vi "crane_pressure_view.vi"() -> ()   [LabVIEW 2024]
panel:
  out "l5_ground_pressure":dbl(slide)
  out "l4_ground_pressure":dbl(slide)
  out "l3_ground_pressure":dbl(slide)
  out "l2_ground_pressure":dbl(slide)
  out "l1_ground_pressure":dbl(slide)
  out "error out":errorcluster
  in  "stop":bool
  out "period(Hz)":dbl(knob) scale=0.0..20.0
  out "l5_gp_max":bool
  out "l4_gp_max":bool
  out "l3_gp_max":bool
  out "l2_gp_max":bool
  out "l1_gp_max":bool
  out "r5_gp_max":bool
  out "r4_gp_max":bool
  out "r3_gp_max":bool
  out "r2_gp_max":bool
  out "r1_gp_max":bool
  out "MaxGroundPressure":dbl(graph)
  out "Load_state":cluster{"Load(kg)":dbl, "Load_Height(m)":dbl}(graph)
  out "Angle":T1(graph)
  in  "Load_Height(m)":dbl(slide) scale=0.0..10.0
  in  "Load(ton)":dbl(slide) scale=1.0..2.0
  in  "boom_angle(degree)":dbl(knob) scale=30.0..50.0
  in  "swing_angle(degree)":dbl(knob) scale=0.0..90.0
  out "r5_ground_pressure":dbl(slide) scale=0.0..10.0
  out "r4_ground_pressure":dbl(slide) scale=0.0..10.0
  out "r3_ground_pressure":dbl(slide) scale=0.0..10.0
  out "r2_ground_pressure":dbl(slide) scale=0.0..10.0
  out "r1_ground_pressure":dbl(slide) scale=0.0..10.0
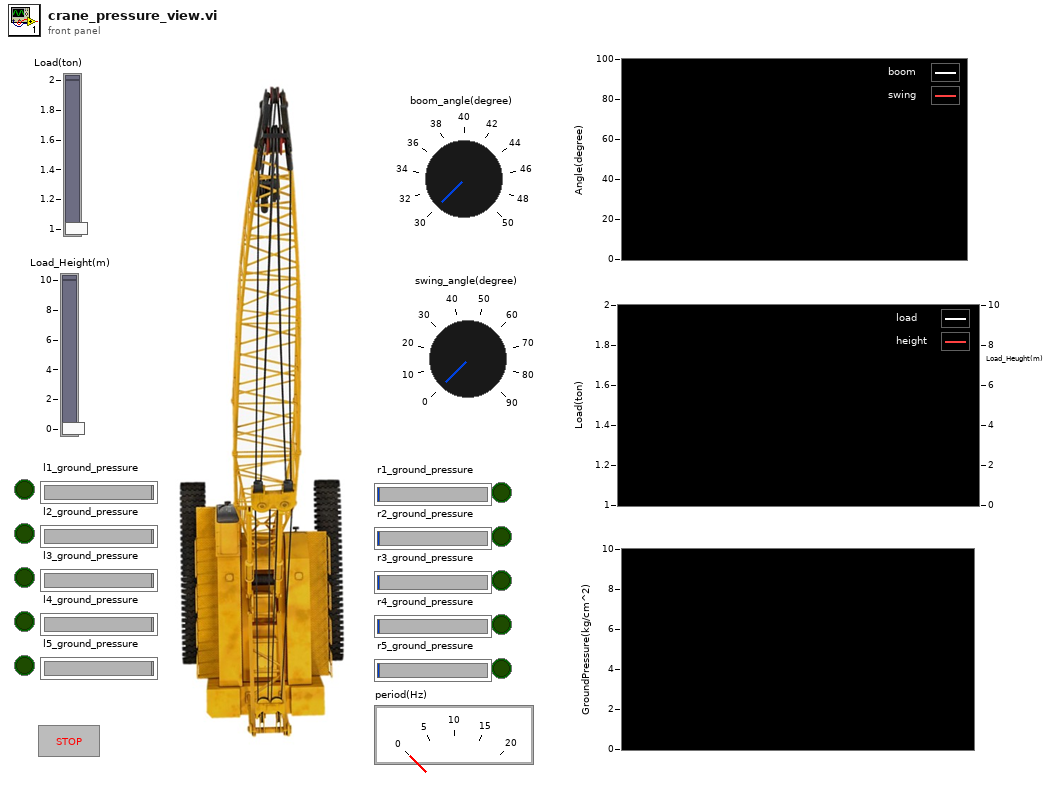
[diagram p1: front panel]
types:
  T1 = cluster{"boom_angle(degree)":dbl, "swing_angle(degree)":dbl}
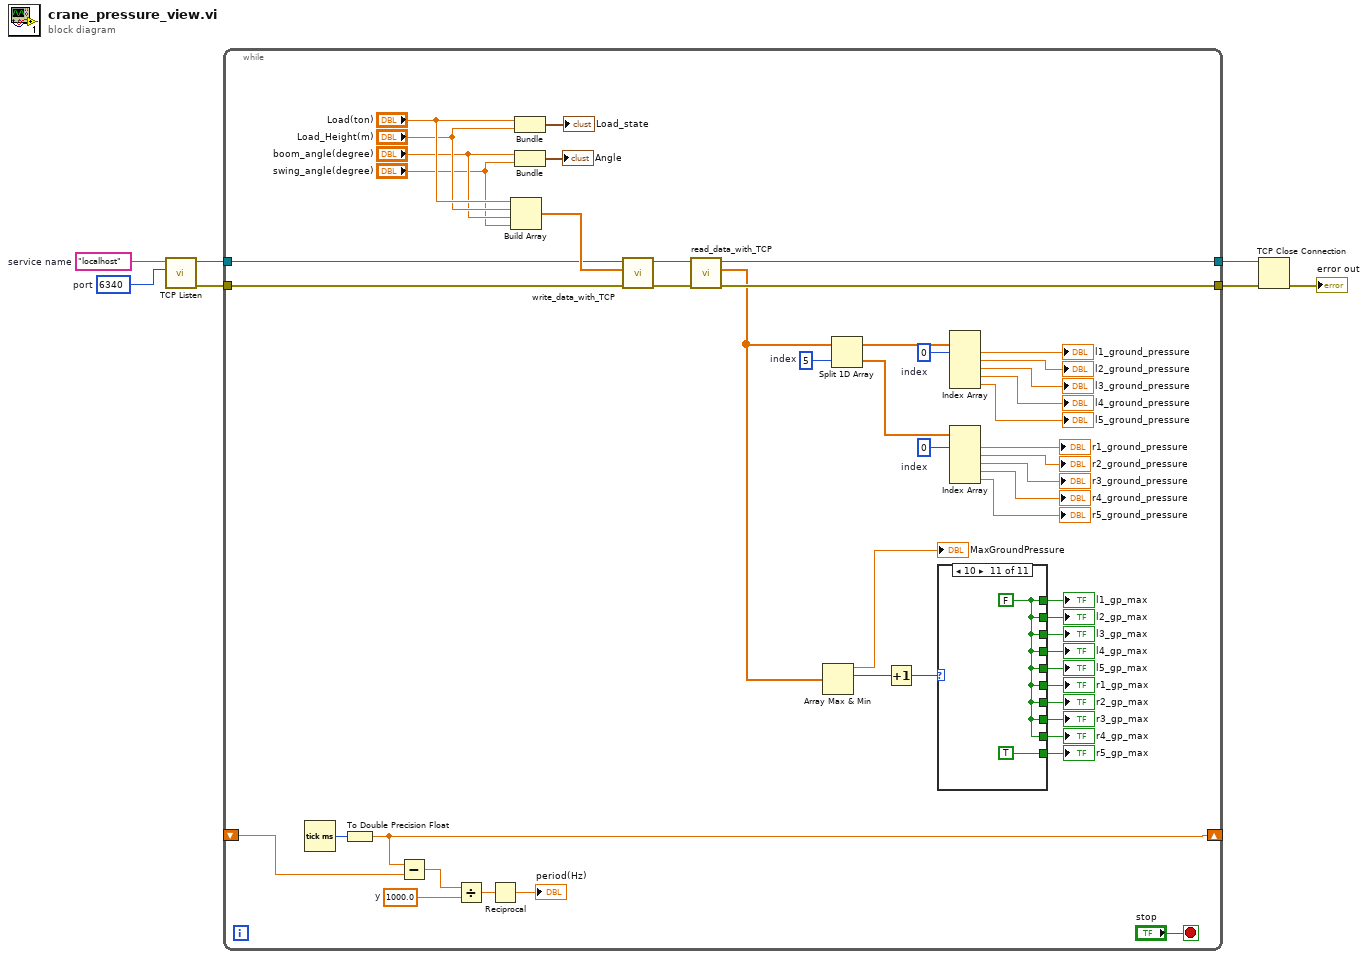
[diagram p0: block diagram]
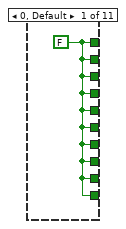
[diagram p2: hidden frame]
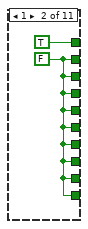
[diagram p3: hidden frame]
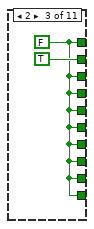
[diagram p4: hidden frame]
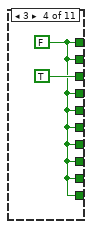
[diagram p5: hidden frame]
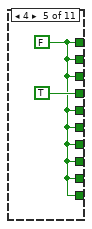
[diagram p6: hidden frame]
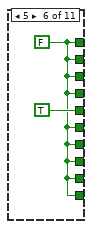
[diagram p7: hidden frame]
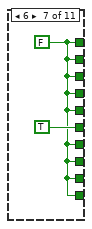
[diagram p8: hidden frame]
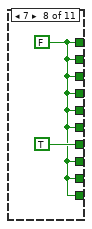
[diagram p9: hidden frame]
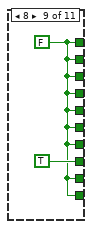
[diagram p10: hidden frame]
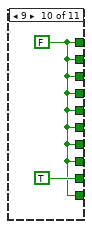
[diagram p11: hidden frame]
diagram:
  w6 = u16 6340  # port
  w7 = "localhost"  # service name
  n1 = call <vilib>:"TCP Listen.vi"("port"=w6, "service name"=w7) -> ("error out"=w4:errorcluster, "connection ID"=w5:refnum<k5>)  [unwired: 5 in, 3 out]
  n2 = while {
    tunnel: w5 -> [w38]
    tunnel: w4 -> [w37]
    tunnel: [w36] -> w3
    tunnel: [w35] -> w2
    shift-right: [w30] -> _
    shift-left: _ -> [w29]
    stop <- "stop" stop-if-true
    w19 = 0  # index
    w21 = 5  # index
    w33 = 1000.0  # y
    w39 = 0  # index
    n3 = Tick Count (ms)() -> (millisecond timer value=w31:u32)
    n4 = To Double Precision Float(number=w31) -> (double precision float=w30:dbl)
    n5 = Subtract(x=w30, y=w29) -> (x-y=w34:dbl)
    n6 = Divide(x=w34, y=w33) -> (x/y=w32:dbl)
    n7 = Reciprocal(x=w32) -> (1/x=→"period(Hz)":dbl)
    n8 = Build Array("Load(ton)", "Load_Height(m)", "boom_angle(degree)", "swing_angle(degree)") -> (w44:dbl[])
    n9 = Bundle("Load(ton)"="Load(ton)", "Load_Height(m)"="Load_Height(m)") -> (→"Load_state":cluster{"Load(ton)":dbl, "Load_Height(m)":dbl})  [unwired: 1 in]
    n10 = Bundle("boom_angle(degree)"="boom_angle(degree)", "swing_angle(degree)"="swing_angle(degree)") -> (→"Angle":T1)  [unwired: 1 in]
    n11 = call "write_data_with_TCP.vi"("error_in"=w37, "data_in"=w44, "TCP_ref_in"=w38) -> ("error_out"=w40:errorcluster, "TCP_ref_out"=w41:refnum<k5>)  [unwired: 7 in]
    n12 = call "read_data_with_TCP.vi"("error_in"=w40, "TCP_ref_in"=w41) -> ("error_out"=w35:errorcluster, "data_out"=w22:dbl[], "TCP_ref_out"=w36:refnum<k5>)  [unwired: 7 in]
    n13 = Array Max & Min(array=w22) -> (max value=→"MaxGroundPressure":dbl, max index (indices)=w47:i32)  [unwired: 2 out]
    n14 = Split 1D Array(array=w22, index=w21) -> (first subarray=w13:dbl[], second subarray=w20:dbl[])
    n15 = Increment(x=w47) -> (x+1=w46:i32)
    n16 = case shown="10" w46 {
      tunnel: [w58 TRUE w61 w63 w65 w67 w69 w71 w73 w75 w77] -> w57
      tunnel: [w58 w59 TRUE w63 w65 w67 w69 w71 w73 w75 w77] -> w56
      tunnel: [w58 w59 w61 TRUE w65 w67 w69 w71 w73 w75 w77] -> w55
      tunnel: [w58 w59 w61 w63 TRUE w67 w69 w71 w73 w75 w77] -> w54
      tunnel: [w58 w59 w61 w63 w65 TRUE w69 w71 w73 w75 w77] -> w53
      tunnel: [w58 w59 w61 w63 w65 w67 TRUE w71 w73 w75 w77] -> w52
      tunnel: [w58 w59 w61 w63 w65 w67 w69 TRUE w73 w75 w77] -> w51
      tunnel: [w58 w59 w61 w63 w65 w67 w69 w71 TRUE w75 w77] -> w50
      tunnel: [w58 w59 w61 w63 w65 w67 w69 w71 w73 TRUE w77] -> w49
      tunnel: [w58 w59 w61 w63 w65 w67 w69 w71 w73 w75 TRUE] -> w48
      frame 0, Default {
        w58 = FALSE
      }
      frame 1 {
        w59 = FALSE
      }
      frame 2 {
        w61 = FALSE
      }
      frame 3 {
        w63 = FALSE
      }
      frame 4 {
        w65 = FALSE
      }
      frame 5 {
        w67 = FALSE
      }
      frame 6 {
        w69 = FALSE
      }
      frame 7 {
        w71 = FALSE
      }
      frame 8 {
        w73 = FALSE
      }
      frame 9 {
        w75 = FALSE
      }
      frame 10 {
        w77 = FALSE
      }
    }
    "r1_gp_max" <- w52
    "r2_gp_max" <- w51
    "r3_gp_max" <- w50
    "r4_gp_max" <- w49
    "r5_gp_max" <- w48
    "l1_gp_max" <- w57
    "l2_gp_max" <- w56
    "l3_gp_max" <- w55
    "l4_gp_max" <- w54
    "l5_gp_max" <- w53
    n17 = Index Array(array=w13, index #1=w39) -> (element #1=→"l1_ground_pressure":dbl, element #2=→"l2_ground_pressure":dbl, element #3=→"l3_ground_pressure":dbl, element #4=→"l4_ground_pressure":dbl, element #5=→"l5_ground_pressure":dbl)  [unwired: 4 in]
    n18 = Index Array(array=w20, index #1=w19) -> (element #1=→"r1_ground_pressure":dbl, element #2=→"r2_ground_pressure":dbl, element #3=→"r3_ground_pressure":dbl, element #4=→"r4_ground_pressure":dbl, element #5=→"r5_ground_pressure":dbl)  [unwired: 4 in]
  }
  n19 = TCP Close Connection(connection ID=w3, error in (no error)=w2) -> (error out=→"error out":errorcluster)  [unwired: 1 in, 1 out]
